vi "NF WF1973_74 FREQ User.vi"(0 "VISAsession":refnum<visa-resource-name>, 2 "Scale(0)":dbl format="%.2f", 3 "Offset(0)":dbl format="%.2f", 5 "Unit Name(DEFA)":string="DEFA", 11 "error in (no error)":errorcluster caption="Error IN", 12 "Read(F)":bool, 13 "Ch(Ch1)":bool) -> (4 "CopyVISAsession":refnum<visa-resource-name>, 6 "Query Unit":string, 15 "error out":errorcluster caption="Error OUT")   [LabVIEW 2010]
panel:
  in  "Type(Linear)":u16(ring) items=["Linear", "Logarithmic"]
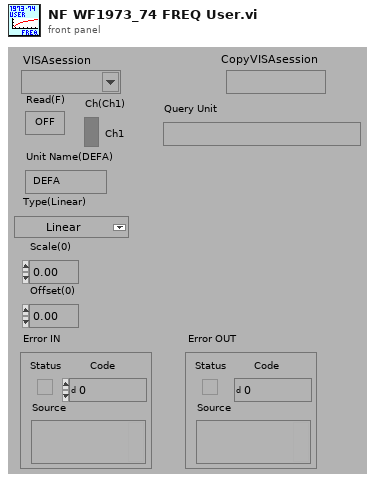
[diagram p1: front panel]
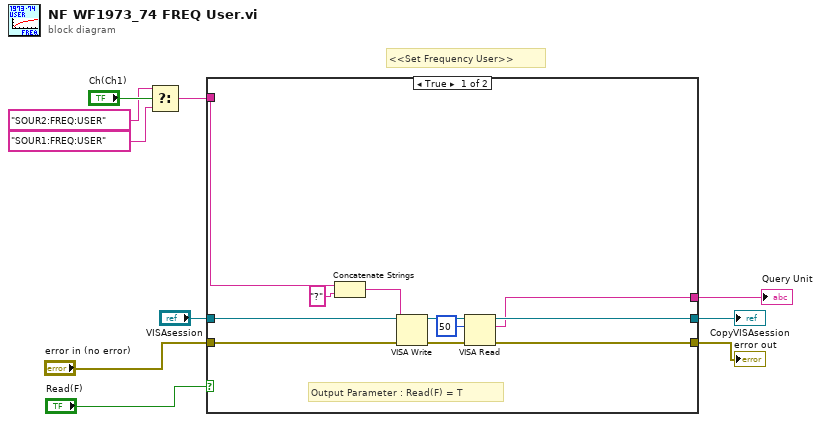
[diagram p0: block diagram]
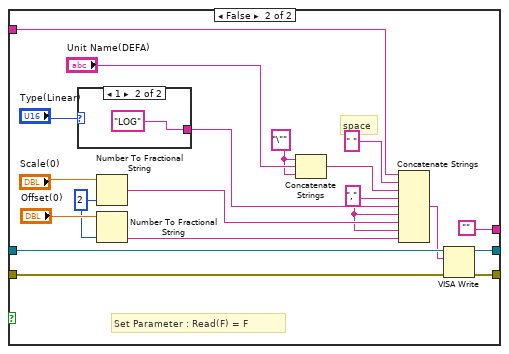
[diagram p2: hidden frame]
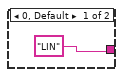
[diagram p3: hidden frame]
diagram:
  # "<<Set Frequency User>>"
  n1 = Select(t="SOUR2:FREQ:USER" ("文字列"), s="Ch(Ch1)", f="SOUR1:FREQ:USER" ("文字列")) -> (s? t:f=w4:string)
  n2 = case shown="TRUE" "Read(F)" {
    tunnel: "VISAsession" -> [w21 w40]
    tunnel: [w18 w38] -> w9
    tunnel: [w17 w39] -> w8
    tunnel: "error in (no error)" -> [w16 w36]
    tunnel: w4 -> [w13 w34]
    tunnel: [w14 ""] -> w1
    frame True {
      # "Output Parameter : Read(F) = T"
      n3 = Concatenate Strings(w13, "?" ("文字列")) -> (w11:string)
      n4 = VISA Write(VISA resource name=w21, write buffer=w11, error in (no error)=w16) -> (VISA resource name out=w19:refnum<visa-resource-name>, error out=w20:errorcluster)  [unwired: 1 out]
      n5 = VISA Read(VISA resource name=w19, byte count=u32 50 ("バイトカウント（0）"), error in (no error)=w20) -> (VISA resource name out=w18:refnum<visa-resource-name>, read buffer=w14:string, error out=w17:errorcluster)  [unwired: 1 out]
    }
    frame False {
      w25 = i16 2 ("精度 (6)")
      w22 = ","
      w31 = "\""
      # "space"
      # "Set Parameter : Read(F) = F"
      n6 = case shown="1" "Type(Linear)" {
        tunnel: ["LIN" "LOG"] -> w23
        frame 0, Default {
        }
        frame 1 {
        }
      }
      n7 = Number To Fractional String(number="Scale(0)", precision (6)=w25) -> (F-format string=w27:string)  [unwired: 2 in]
      n8 = Number To Fractional String(number="Offset(0)", precision (6)=w25) -> (F-format string=w26:string)  [unwired: 2 in]
      n9 = Concatenate Strings(w31, "Unit Name(DEFA)", w31) -> (w30:string)
      n10 = Concatenate Strings(w34, " ", w30, w22, w23, w22, w27, w22, w26) -> (w37:string)
      n11 = VISA Write(VISA resource name=w40, write buffer=w37, error in (no error)=w36) -> (VISA resource name out=w38:refnum<visa-resource-name>, error out=w39:errorcluster)  [unwired: 1 out]
    }
  }
  "error out" <- w8
  "CopyVISAsession" <- w9
  "Query Unit" <- w1
